vi "Dodanie punktu do listy punkty na podstawie współrzędnych geograficznych.vi"(7 "Nazwa punktu":string, 9 "UTM":T1, 10 "Współrzędne punktu":string, 11 "Lista współrzędnych":string[][](array[string])) -> (3 "output array":string[][](array[string]))   [LabVIEW 2012, in "Biblioteka moduł map v3.lvlib" / "Obsługa listy współrzędnych.lvlib"]
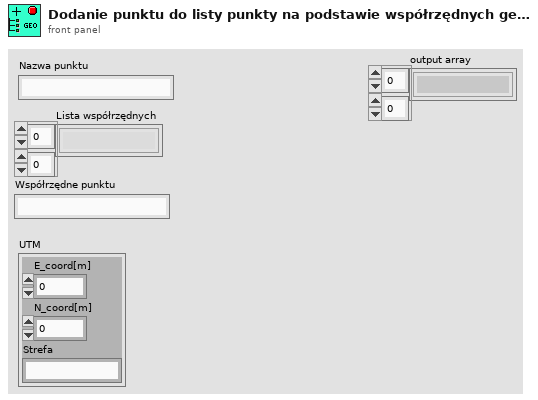
[diagram p1: front panel]
types:
  T1 = cluster{"E_coord[m]":ext, "N_coord[m]":ext, "Strefa":string}
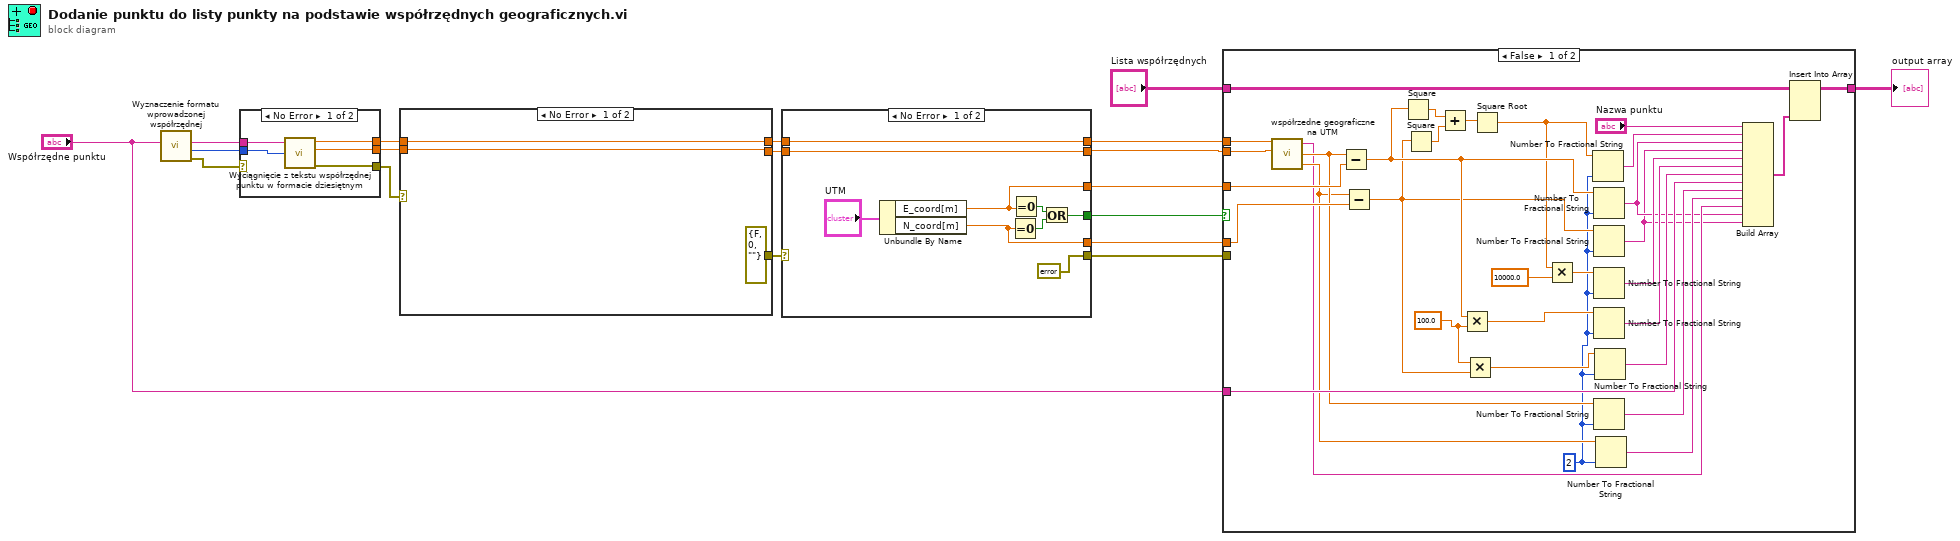
[diagram p0: block diagram]
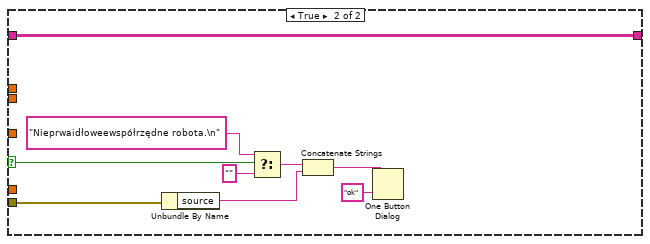
[diagram p2: hidden frame]
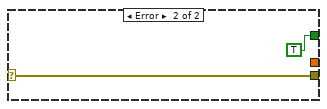
[diagram p3: hidden frame]
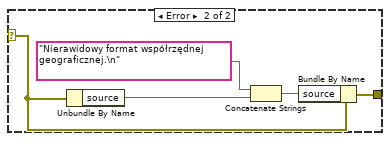
[diagram p4: hidden frame]
diagram:
  n1 = call "Wyznaczenie formatu wprowadzonej współrzędnej.vi"("Współrzędna geograficzna"="Współrzędne punktu") -> ("error constant"=w13:errorcluster, "Format wprowadzonej współrzędnej"=w14:i32, "Znaleziony tekst"=w15:string)  [unwired: 8 in]
  n2 = case shown="No Error" w13 {
    selector: w13 -> [_ w24]
    tunnel: w15 -> [w23 _]
    tunnel: w14 -> [w22 _]
    tunnel: [w21 _] -> w17
    tunnel: [w20 _] -> w18
    tunnel: [w19 w24] -> w16
    frame No Error {
      n3 = call "Wyciągnięcie z tekstu współrzędnej punktu w formacie dziesiętnym.vi"("Format wprowadzanej współrzędnej"=w22, "Współrzędna w postaci tekstowej"=w23) -> ("error constant"=w19:errorcluster, "Szerokość geograficzna (NS)"=w20:dbl, "Długość geograficzna (EW)"=w21:dbl)  [unwired: 4 in]
    }
    frame Error {
    }
  }
  n4 = case shown="No Error" w16 {
    selector: w16 -> [_ w30]
    tunnel: [errorcluster {"status"=FALSE, "code"=0, "source"=""} ("error IO") w29] -> w12
    tunnel: w17 -> [w27 _]
    tunnel: w18 -> [w26 _]
    tunnel: [w27 _] -> w4
    tunnel: [w26 _] -> w3
    frame No Error {
    }
    frame Error {
      n5 = Unbundle By Name(w30) -> ("source"=w31:string)
      n6 = Concatenate Strings("Nierawidowy format współrzędnej geograficznej.\n" ("message"), w31) -> (w28:string)
      n7 = Bundle By Name(cluster=w30, "source"=w28) -> (w29:errorcluster)
    }
  }
  n8 = case shown="No Error" w12 {
    selector: w12 -> [_ w42]
    tunnel: [w39 TRUE] -> w11
    tunnel: [errorcluster {"status"=FALSE, "code"=0, "source"=""} ("error IO") w42] -> w10
    tunnel: [w33 _] -> w7
    tunnel: [w34 _] -> w6
    tunnel: [w37 _] -> w5
    tunnel: w4 -> [w37 _]
    tunnel: [w36 _] -> w2
    tunnel: w3 -> [w36 _]
    frame No Error {
      n9 = Unbundle By Name("UTM") -> ("E_coord[m]"=w34:ext, "N_coord[m]"=w33:ext)
      n10 = Equal To 0?(x=w33) -> (x = 0?=w40:bool)
      n11 = Equal To 0?(x=w34) -> (x = 0?=w41:bool)
      n12 = Or(x=w41, y=w40) -> (x .or. y?=w39:bool)
    }
    frame Error {
    }
  }
  n13 = case shown="False" w11 {
    selector: w11 -> [_ w82]
    tunnel: w10 -> [_ w84]
    tunnel: [w75 w76] -> w9
    tunnel: "Lista współrzędnych" -> [w74 w76]
    tunnel: w7 -> [w68 _]
    tunnel: w6 -> [w69 _]
    tunnel: w5 -> [w71 _]
    tunnel: w2 -> [w70 _]
    tunnel: "Współrzędne punktu" -> [w52 _]
    frame False {
      w44 = i16 2 ("precision (6)")
      w67 = 100.0 ("y")
      n14 = call "współrzedne geograficzne na UTM.vi"("Położenie robota - długość geograficzna"=w71, "Położenie robota - szerokość geograficzna"=w70) -> ("Strefa"=w47:string, "E"=w51:ext, "N"=w50:ext)  [unwired: 4 in]
      n15 = Subtract(x=w51, y=w69) -> (x-y=w60:ext)
      n16 = Subtract(x=w50, y=w68) -> (x-y=w59:ext)
      n17 = Square(x=w60) -> (x^2=w62:ext)
      n18 = Square(x=w59) -> (x^2=w63:ext)
      n19 = Add(x=w62, y=w63) -> (x+y=w64:ext)
      n20 = Multiply(x=w60, y=w67) -> (x*y=w66:ext)
      n21 = Multiply(x=w67, y=w59) -> (x*y=w65:ext)
      n22 = Square Root(x=w64) -> (sqrt(x)=w57:ext)
      n23 = Multiply(x=w57, y=10000.0) -> (x*y=w56:ext)
      n24 = Number To Fractional String(number=w57, precision (6)=w44) -> (F-format string=w61:string)  [unwired: 2 in]
      n25 = Number To Fractional String(number=w60, precision (6)=w44) -> (F-format string=w46:string)  [unwired: 2 in]
      n26 = Number To Fractional String(number=w59, precision (6)=w44) -> (F-format string=w45:string)  [unwired: 2 in]
      n27 = Number To Fractional String(number=w56, precision (6)=w44) -> (F-format string=w55:string)  [unwired: 2 in]
      n28 = Number To Fractional String(number=w66, precision (6)=w44) -> (F-format string=w54:string)  [unwired: 2 in]
      n29 = Number To Fractional String(number=w51, precision (6)=w44) -> (F-format string=w49:string)  [unwired: 2 in]
      n30 = Number To Fractional String(number=w65, precision (6)=w44) -> (F-format string=w53:string)  [unwired: 2 in]
      n31 = Number To Fractional String(number=w50, precision (6)=w44) -> (F-format string=w48:string)  [unwired: 2 in]
      n32 = Build Array("Nazwa punktu", w61, w46, w45, w55, w54, w53, w52, w49, w48, w47, w46, w45) -> (w72:string[])
      n33 = Insert Into Array(array=w74, new element=w72) -> (w75:string[][])  [unwired: 2 in]
    }
    frame True {
      n34 = Unbundle By Name(w84) -> ("source"=w78:string)
      n35 = Select(t="Nieprwaidłoweewspółrzędne robota.\n" ("button name (\"OK\")"), s=w82, f="") -> (s? t:f=w79:string)
      n36 = Concatenate Strings(w79, w78) -> (w77:string)
      n37 = One Button Dialog(message=w77, button name ("OK")="ok") -> ()  [unwired: 1 out]
    }
  }
  "output array" <- w9
